vi "planing.vi"() -> ()   [LabVIEW 2020]
panel:
  out "*(type *) &x 2":string
  out "String":string
  out "*(type *) &x":u8[](array[numeric])
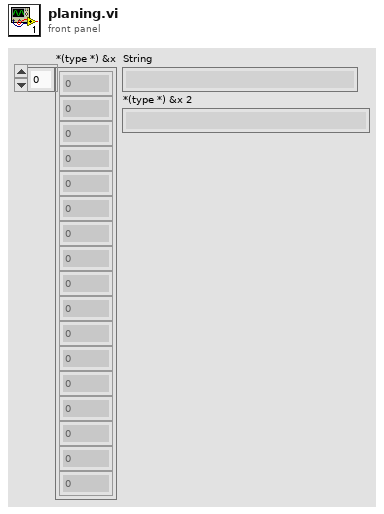
[diagram p1: front panel]
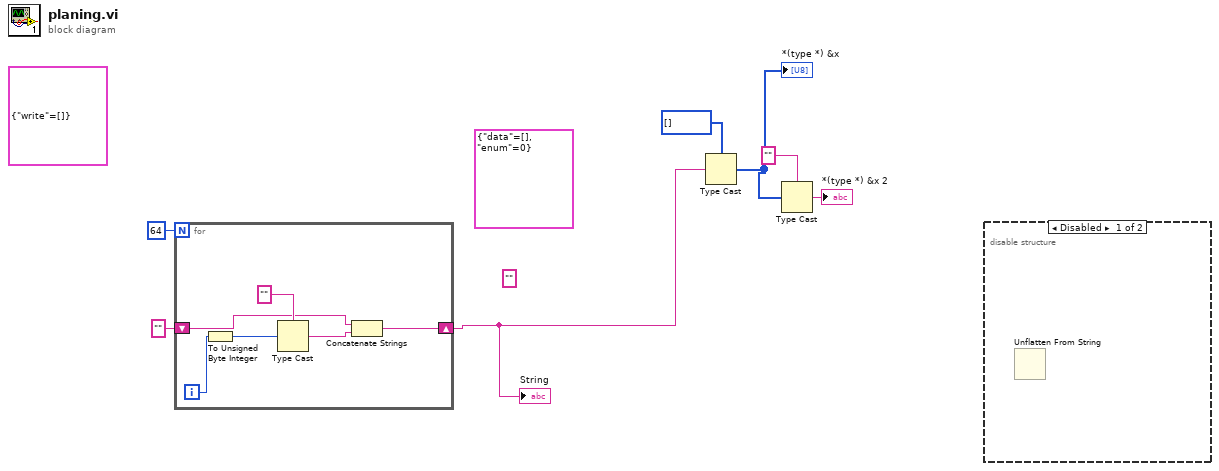
[diagram p0: block diagram]
diagram:
  (unwired) cluster{"write":u8[]} {"write"=[]}
  (unwired) ""
  (unwired) cluster{"data":u8[], "enum":u8} {"data"=[], "enum"=0}
  n1 = for {
    N: 64 -> [_]
    shift-right: [w10] -> w4
    shift-left: "" -> [w9]
    i -> [w13]
    n2 = To Unsigned Byte Integer(number=w13) -> (unsigned 8bit integer=w8:u8)
    n3 = Type Cast(type="", x=w8) -> (*(type *) &x=w11:string)
    n4 = Concatenate Strings(w9, w11) -> (w10:string)
  }
  "String" <- w4
  n5 = Type Cast(type=u8[] [], x=w4) -> (*(type *) &x=w3:u8[])
  "*(type *) &x" <- w3
  n6 = Type Cast(type="", x=w3) -> (*(type *) &x=→"*(type *) &x 2":string)
  n7 = disable-structure shown="Disabled" {
    frame Disabled {
      n8 = Unflatten From String() -> ()  [unwired: 5 in, 3 out]
    }
    frame Enabled {
    }
  }
